vi "Client.vi"() -> ()   [LabVIEW 2019]
uses:
  padrao_tipo_dado.ctl
  padrao_todos_os_dados_ENTRADA.ctl
  padrao_UCM.004.EEL.0300_ENTRADA.ctl
  padrao_UCM.004.EEL.0200_ENTRADA.ctl
  padrao_INTERNO.ctl
  padrao_todos_os_dados_SAIDA.ctl
  padrao_UCM.004.EEL.0300_SAIDA.ctl
  padrao_UCM.004.EEL.0200_SAIDA.ctl
  padrao_enum.ctl
  padrao_TAGS_prioridades_client.ctl
  padrao_dados_cliente_para_server.ctl
  padrao_informacoes_meu_computador.ctl
  <vilib>/Utility/config.llb/NI_LVConfig.lvlib
panel:
  out "Array_TAGS":string[](array[string])
  in  "todos_os_dados_SAIDA":T1
  out "todos_os_dados_ENTRADA":T5
  in  "TAG_para_PDF":string
  in  "Refresh Button":bool
  in  "Seleciona_variaveis_prioridade":bool
  in  "Tipo de Dado":T8 items=["Engenharia", "Puro(mA)"]
  out "Nome_meu_computador":string
  out "Meu IP":string
  out "Status_Comunicação":string
  out "led_indica_comunicacao":bool
  in  "Endereço IP do Server":string(combo)
  in  "[ESC]":bool
  out "Erro":errorcluster
  # "CLIENT"
  # "1) Certifique-se que esse não é o PC Server: Caso for, essa VI não pode rodar nesse computador.\n2) Certifique-se que o Server já esteja rodando:  Caso esteja, você poder rodar essa VI apertando Ctrl+R ou na seta ->\n3) Se não ocorrer nenhum erro, o LED azul irá acender\n4) Coloque o nome do PC caso esteja em branco.\n5) Caso deseje encerrar aperte ESC ou no botão STOP"
  # "Comunicação Via TCP/IP"
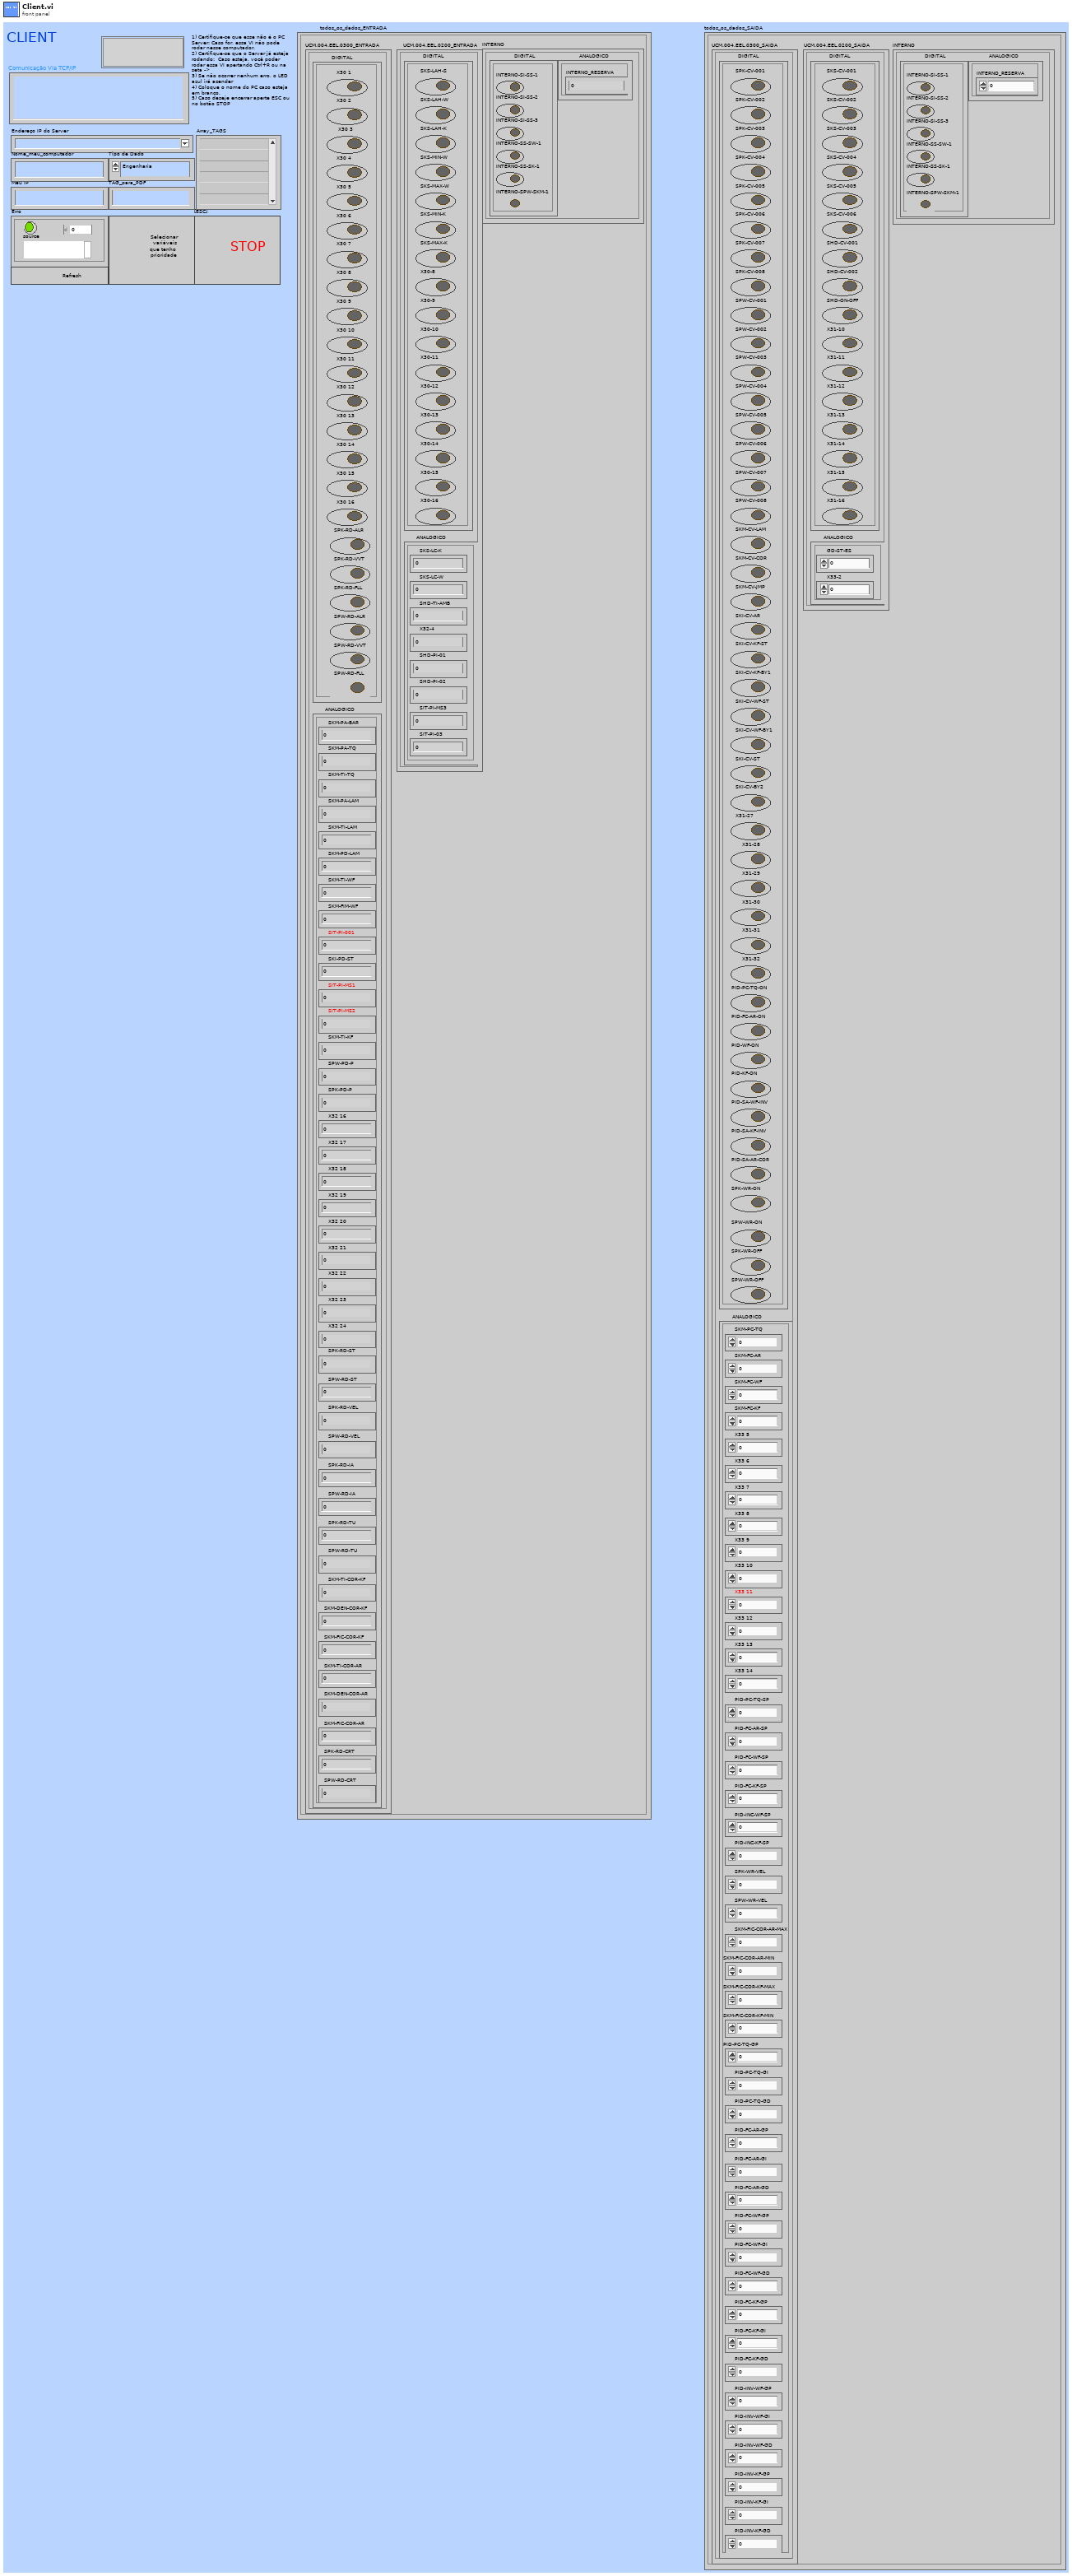
[diagram p1: front panel]
types:
  T1 = typedef "padrao_todos_os_dados_SAIDA.ctl" = cluster{"UCM.004.EEL.0300_SAIDA":T2, "UCM.004.EEL.0200_SAIDA":T3, "INTERNO":T4}
  T2 = typedef "padrao_UCM.004.EEL.0300_SAIDA.ctl" = cluster{"DIGITAL":cluster{"SPK-CV-001":bool, "SPK-CV-002":bool, "SPK-CV-003":bool, "SPK-CV-004":bool, "SPK-CV-005":bool, "SPK-CV-006":bool, "SPK-CV-007":bool, "SPK-CV-008":bool, "SPW-CV-001":bool, "SPW-CV-002":bool, "SPW-CV-003":bool, "SPW-CV-004":bool, "SPW-CV-005":bool, "SPW-CV-006":bool, "SPW-CV-007":bool, "SPW-CV-008":bool, "SKM-CV-LAM":bool, "SKM-CV-COR":bool, "SKM-CV-JMP":bool, "SKI-CV-AR":bool, "SKI-CV-KF-ST":bool, "SKI-CV-KF-BY1":bool, "SKI-CV-WF-ST":bool, "SKI-CV-WF-BY1":bool, "SKI-CV-ST":bool, "SKI-CV-BY2":bool, "X31-27":bool, "X31-28":bool, "X31-29":bool, "X31-30":bool, "X31-31":bool, "X31-32":bool, "PID-PC-TQ-ON":bool, "PID-FC-AR-ON":bool, "PID-WF-ON":bool, "PID-KF-ON":bool, "PID-SA-WF-INV":bool, "PID-SA-KF-INV":bool, "PID-SA-AR-COR":bool, "SPK-WR-ON":bool, "SPW-WR-ON":bool, "SPK-WR-OFF":bool, "SPW-WR-OFF":bool}, "ANALOGICO":cluster{"SKM-PC-TQ":i16, "SKM-FC-AR":i16, "SKM-FC-WF":i16, "SKM-FC-KF":i16, "X33 5":i16, "X33 6":i16, "X33 7":i16, "X33 8":i16, "X33 9":i16, "X33 10":i16, "X33 11":i16, "X33 12":i16, "X33 13":i16, "X33 14":i16, "PID-PC-TQ-SP":i16, "PID-FC-AR-SP":i16, "PID-FC-WF-SP":i16, "PID-FC-KF-SP":i16, "PID-INC-WF-SP":i16, "PID-INC-KF-SP":i16, "SPK-WR-VEL":i32, "SPW-WR-VEL":i32, "SKM-FIC-COR-AR-MAX":dbl, "SKM-FIC-COR-AR-MIN":dbl, "SKM-FIC-COR-KF-MAX":dbl, "SKM-FIC-COR-KF-MIN":dbl, "PID-PC-TQ-GP":dbl, "PID-PC-TQ-GI":dbl, "PID-PC-TQ-GD":dbl, "PID-FC-AR-GP":dbl, "PID-FC-AR-GI":dbl, "PID-FC-AR-GD":dbl, "PID-FC-WF-GP":dbl, "PID-FC-WF-GI":dbl, "PID-FC-WF-GD":dbl, "PID-FC-KF-GP":dbl, "PID-FC-KF-GI":dbl, "PID-FC-KF-GD":dbl, "PID-INV-WF-GP":dbl, "PID-INV-WF-GI":dbl, "PID-INV-WF-GD":dbl, "PID-INV-KF-GP":dbl, "PID-INV-KF-GI":dbl, "PID-INV-KF-GD":dbl}}
  T3 = typedef "padrao_UCM.004.EEL.0200_SAIDA.ctl" = cluster{"DIGITAL":cluster{"SKS-CV-001":bool, "SKS-CV-002":bool, "SKS-CV-003":bool, "SKS-CV-004":bool, "SKS-CV-005":bool, "SKS-CV-006":bool, "SHD-CV-001":bool, "SHD-CV-002":bool, "SHD-ON-OFF":bool, "X31-10":bool, "X31-11":bool, "X31-12":bool, "X31-13":bool, "X31-14":bool, "X31-15":bool, "X31-16":bool}, "ANALOGICO":cluster{"GD-ST-ES":i16, "X33-2":i16}}
  T4 = typedef "padrao_INTERNO.ctl" = cluster{"DIGITAL":cluster{"INTERNO-SI-SS-1":bool, "INTERNO-SI-SS-2":bool, "INTERNO-SI-SS-3":bool, "INTERNO-SS-SW-1":bool, "INTERNO-SS-SK-1":bool, "INTERNO-SPW-SKM-1":bool}, "ANALOGICO":cluster{"INTERNO_RESERVA":dbl}}
  T5 = typedef "padrao_todos_os_dados_ENTRADA.ctl" = cluster{"UCM.004.EEL.0300_ENTRADA":T6, "UCM.004.EEL.0200_ENTRADA":T7, "INTERNO":T4}
  T6 = typedef "padrao_UCM.004.EEL.0300_ENTRADA.ctl" = cluster{"DIGITAL":cluster{"X30 1":bool, "X30 2":bool, "X30 3":bool, "X30 4":bool, "X30 5":bool, "X30 6":bool, "X30 7":bool, "X30 8":bool, "X30 9":bool, "X30 10":bool, "X30 11":bool, "X30 12":bool, "X30 13":bool, "X30 14":bool, "X30 15":bool, "X30 16":bool, "SPK-RD-ALR":bool, "SPK-RD-VVT":bool, "SPK-RD-FLL":bool, "SPW-RD-ALR":bool, "SPW-RD-VVT":bool, "SPW-RD-FLL":bool}, "ANALOGICO":cluster{"SKM-PA-BAR":i16, "SKM-PA-TQ":i16, "SKM-TI-TQ":i16, "SKM-PA-LAM":i16, "SKM-TI-LAM":i16, "SKM-PD-LAM":i16, "SKM-TI-WF":i16, "SKM-FIM-WF":i16, "SIT-PI-001":i16, "SKI-PD-ST":i16, "SIT-PI-MS1":i16, "SIT-PI-MS2":i16, "SKM-TI-KF":i16, "SPW-PD-P":i16, "SPK-PD-P":i16, "X32 16 ":i16, "X32 17":i16, "X32 18":i16, "X32 19":i16, "X32 20":i16, "X32 21":i16, "X32 22":i16, "X32 23":i16, "X32 24":i16, "SPK-RD-ST":i32, "SPW-RD-ST":i32, "SPK-RD-VEL":i32, "SPW-RD-VEL":i32, "SPK-RD-IA":i32, "SPW-RD-IA":i32, "SPK-RD-TU":i32, "SPW-RD-TU":i32, "SKM-TI-COR-KF":dbl, "SKM-DEN-COR-KF":dbl, "SKM-FIC-COR-KF":dbl, "SKM-TI-COR-AR":dbl, "SKM-DEN-COR-AR":dbl, "SPK-RD-CRT":dbl, "SPW-RD-CRT":dbl, "SKM-FIC-COR-AR":dbl}}
  T7 = typedef "padrao_UCM.004.EEL.0200_ENTRADA.ctl" = cluster{"DIGITAL":cluster{"SKS-LAH-S":bool, "SKS-LAH-W":bool, "SKS-LAH-K":bool, "SKS-MIN-W":bool, "SKS-MAX-W":bool, "SKS-MIN-K":bool, "SKS-MAX-K":bool, "X30-8":bool, "X30-9":bool, "X30-10":bool, "X30-11":bool, "X30-12":bool, "X30-13":bool, "X30-14":bool, "X30-15":bool, "X30-16":bool}, "ANALOGICO":cluster{"SKS-LC-K":i16, "SKS-LC-W":i16, "SHD-TI-AMB":i16, "X32-4":i16, "SHD-PI-01":i16, "SHD-PI-02":i16, "SIT-PI-MS3":i16, "SIT-PI-03":i16}}
  T8 = typedef "padrao_tipo_dado.ctl" = u16
  T9 = typedef "padrao_TAGS_prioridades_client.ctl" = cluster{"TAG":string, "Tenho\nPrioridade?":bool}[]
  T10 = typedef "padrao_enum.ctl" = enum16{"open-conection ", "data", "check-status", "Inicio"}
  T11 = typedef "NI_LVConfig.lvlib/Config Data RefNum.ctl" = refnum<k1>
  T12 = typedef "padrao_informacoes_meu_computador.ctl" = cluster{"Nome_computador":string, "IP_meu_computador":string, "Tipo de Dado":T8}
  T13 = typedef "padrao_dados_cliente_para_server.ctl" = cluster{"todos_os_dados_saida":T1, "informacoes_meu_PC":T12, "padrao_prioridade_TAGs":T9}
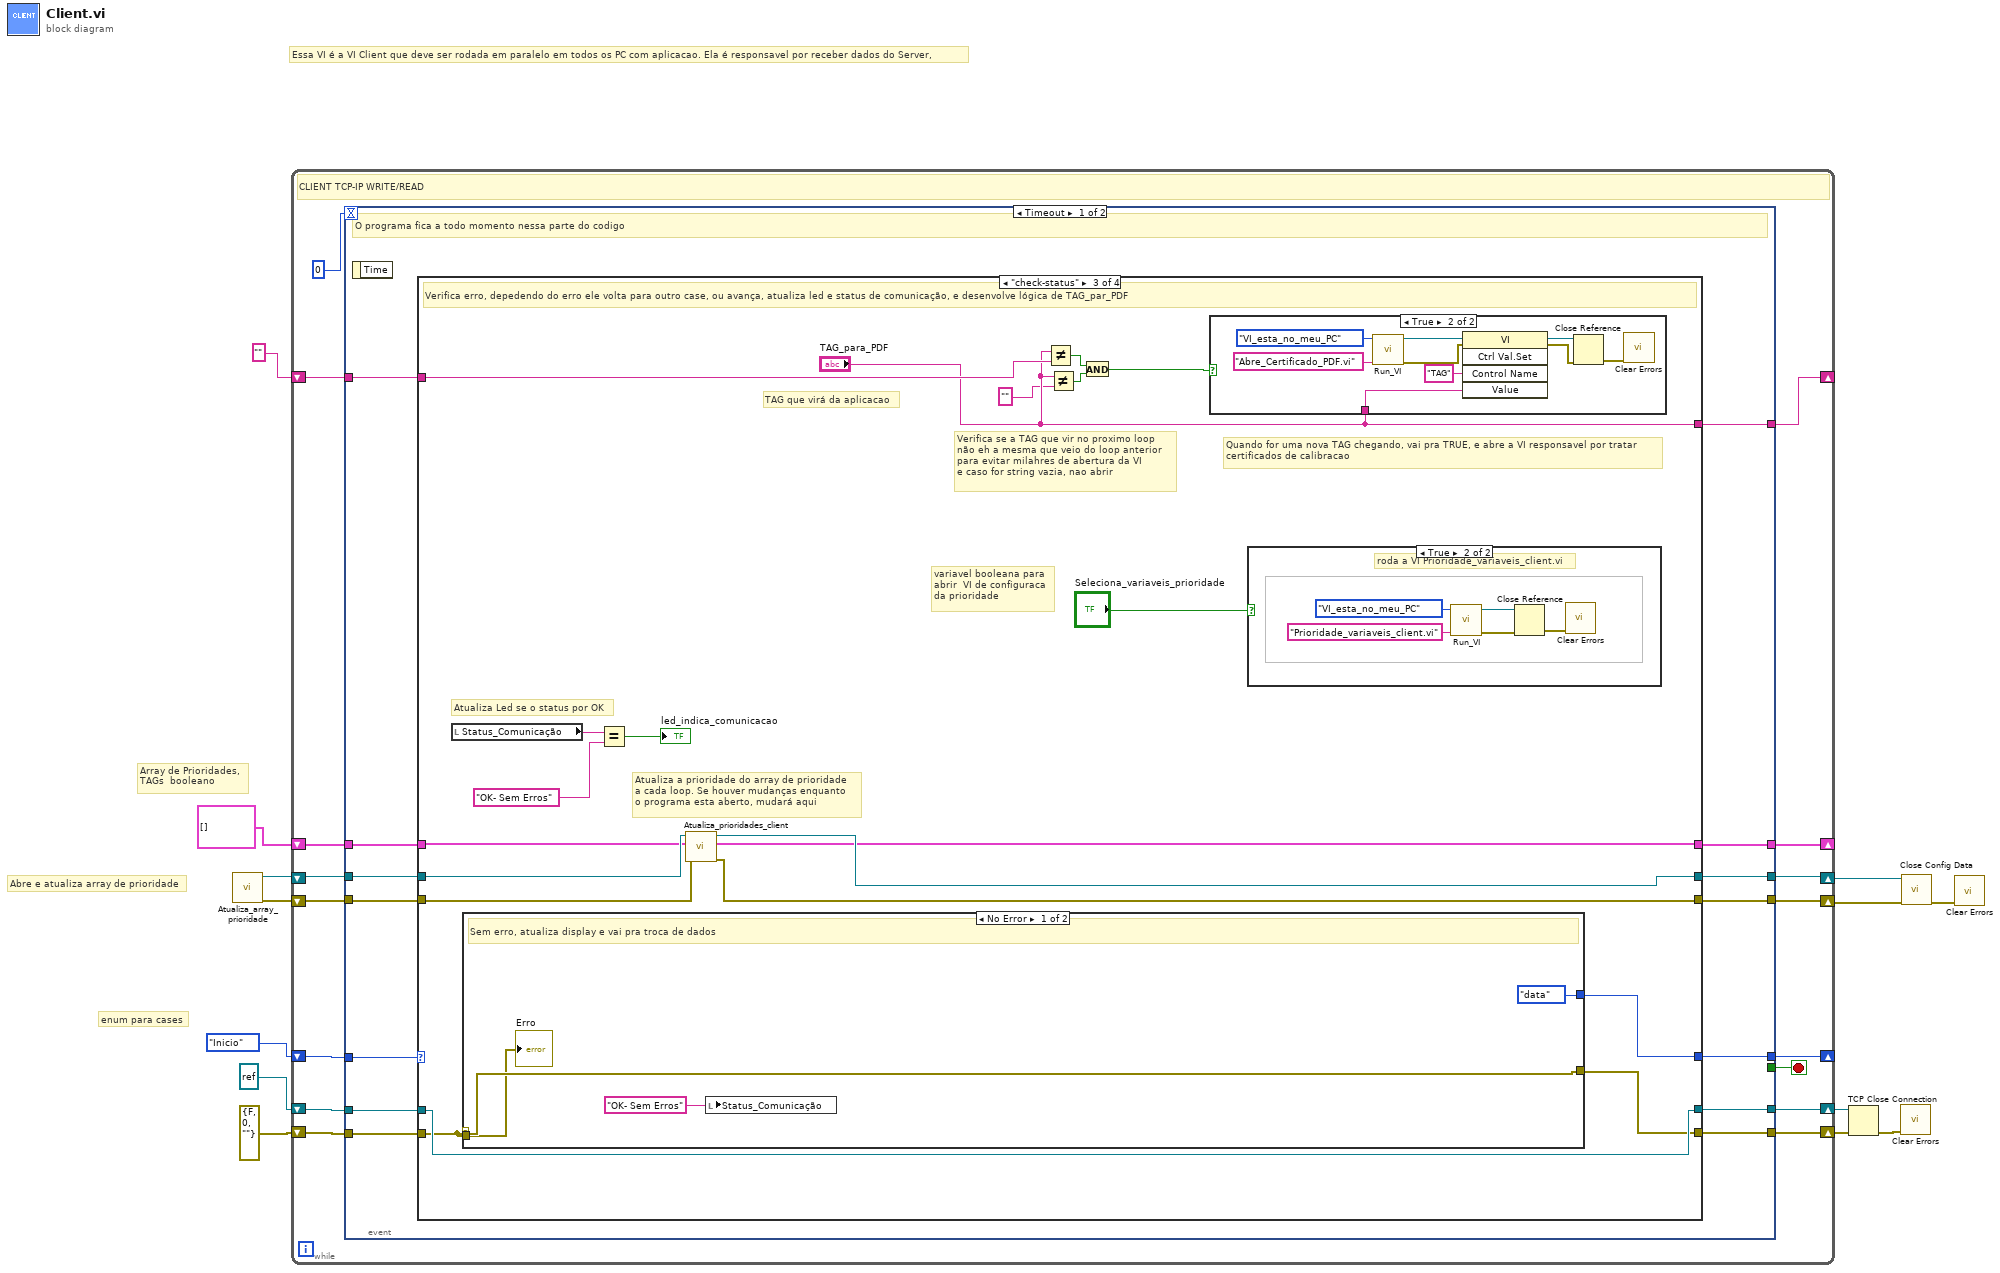
[diagram p0: block diagram]
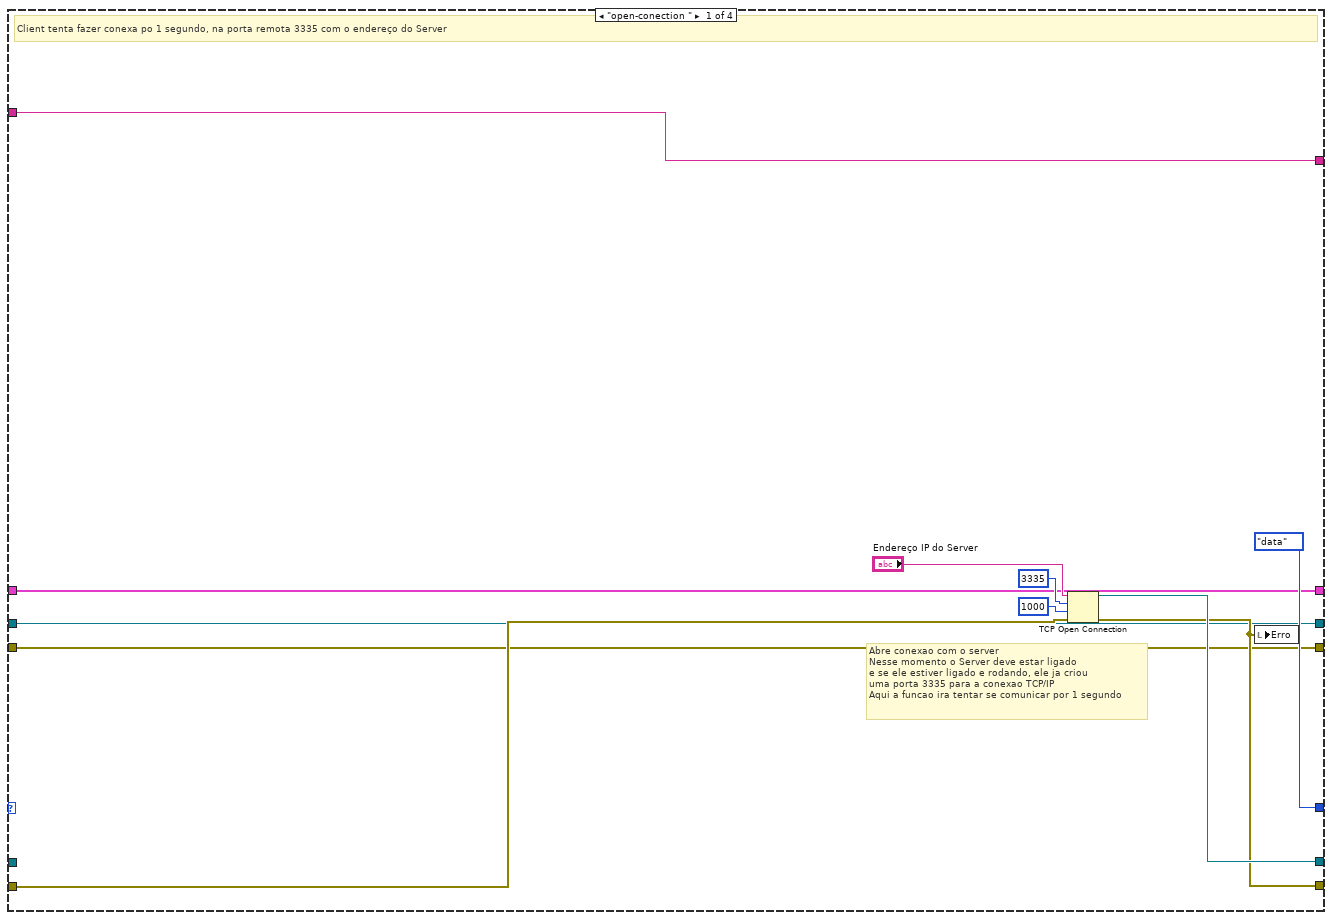
[diagram p2: hidden frame]
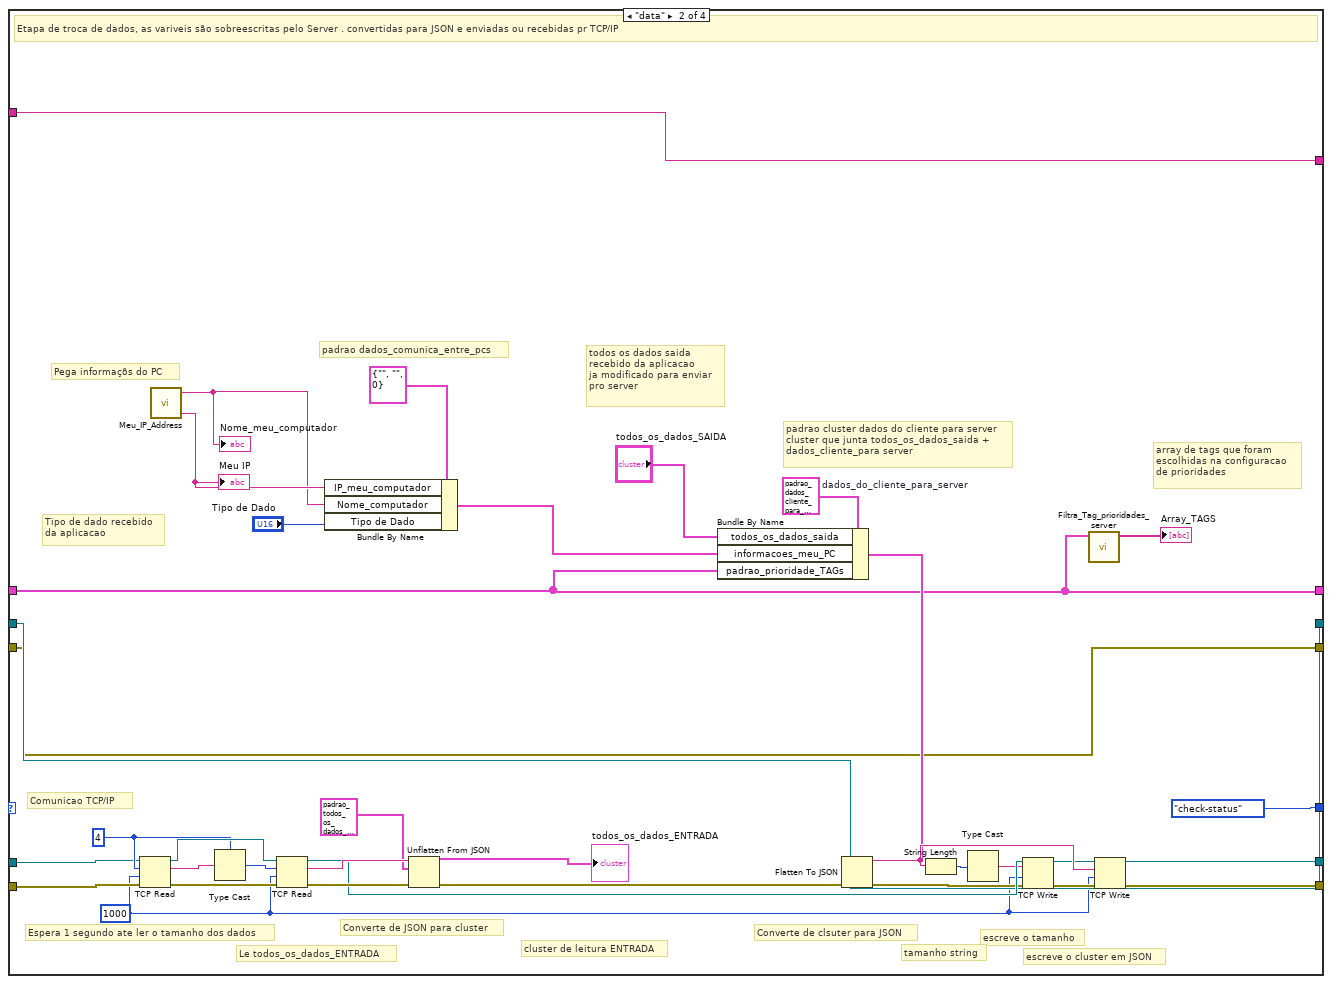
[diagram p3: hidden frame]
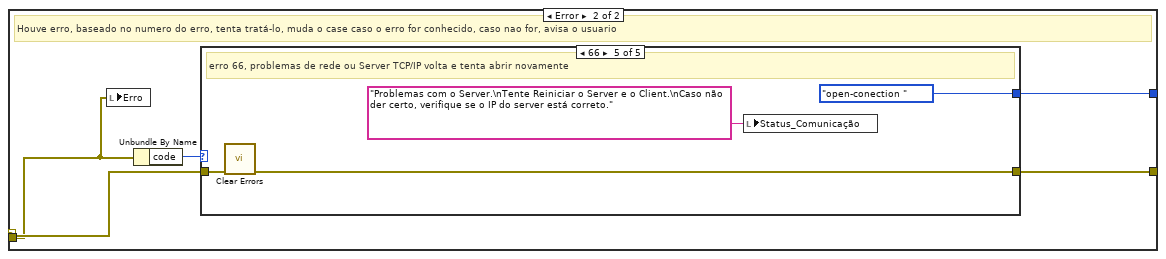
[diagram p6: hidden frame]
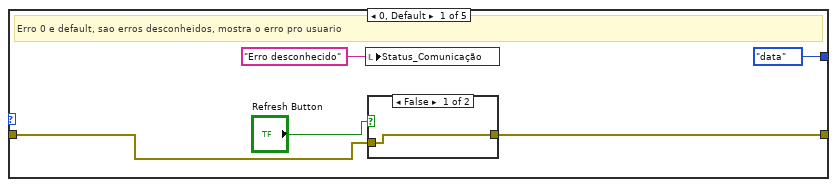
[diagram p7: hidden frame]
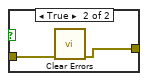
[diagram p8: hidden frame]
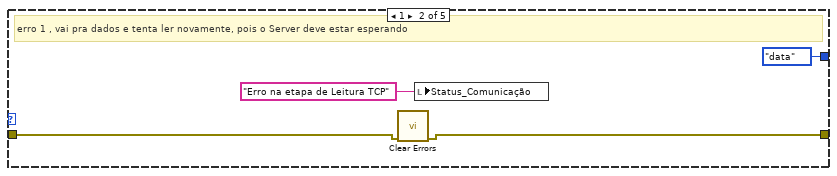
[diagram p9: hidden frame]
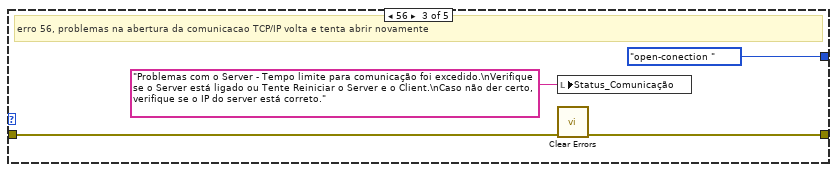
[diagram p10: hidden frame]
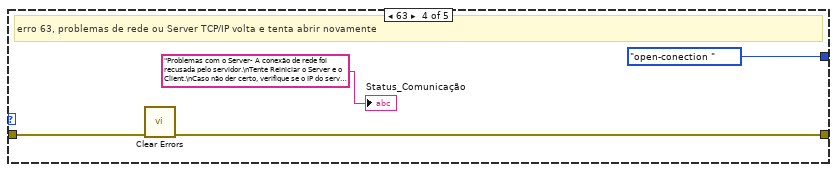
[diagram p11: hidden frame]
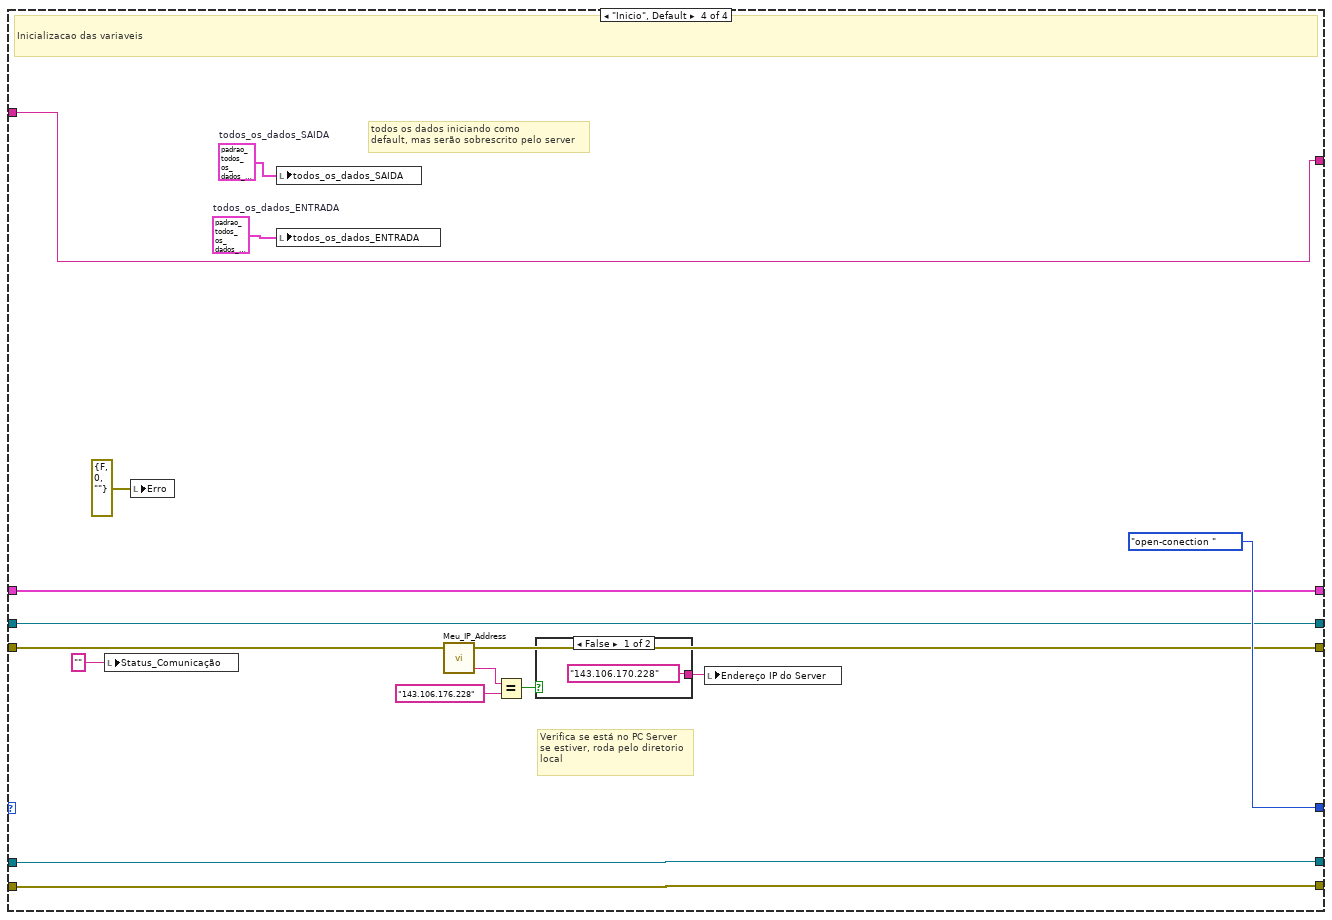
[diagram p12: hidden frame]
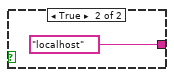
[diagram p13: hidden frame]
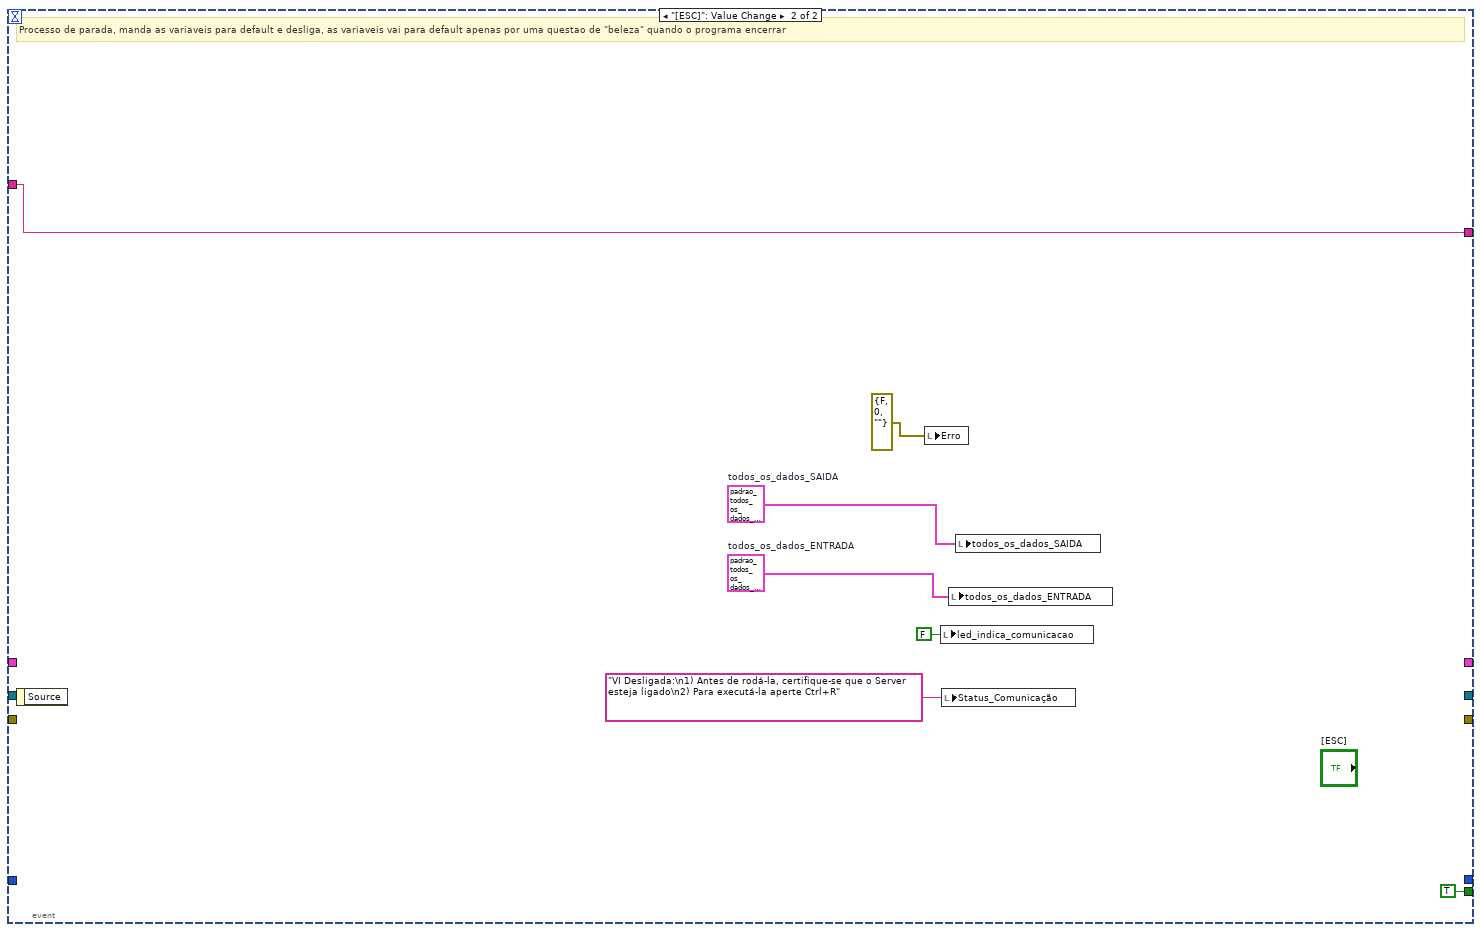
[diagram p14: hidden frame]
diagram:
  # "Array de Prioridades,\nTAGs  booleano"
  # "enum para cases"
  # "Abre e atualiza array de prioridade"
  # "Essa VI é a VI Client que deve ser rodada em paralelo em todos os PC com aplicacao. Ela é responsavel por receber dados do Server,"
  n1 = call "Atualiza_array_prioridade.vi"() -> ("error out"=w1:errorcluster, "refnum"=w2:T11)  [unwired: 10 in]
  n2 = while {
    shift-right: [w26] -> w9
    shift-left: errorcluster {"status"=FALSE, "code"=0, "source"=""} ("error constant") -> [w27]
    shift-right: [w28] -> _
    shift-left: padrao_enum."Inicio" ("Enum") -> [w29]
    shift-right: [w25] -> w10
    shift-left: refnum<k5> refnum ("connection ID") -> [w24]
    shift-right: [w19] -> w6
    shift-left: w2 -> [w21]
    shift-right: [w18] -> w7
    shift-left: w1 -> [w20]
    shift-right: [w16] -> _
    shift-left: T9 [] ("padrao_prioridade_TAGs") -> [w17]
    shift-right: [w14] -> _
    shift-left: "" ("y") -> [w15]
    stop <- w22 stop-if-true
    # "CLIENT TCP-IP WRITE/READ"
    n3 = event shown="[0] Timeout" {
      selector: _ -> [_ _]
      dyn-events: _ -> [_ _]
      timeout: 0 -> [_ _]
      tunnel: w29 -> [w43 _]
      tunnel: [w42 _] -> w28
      tunnel: w27 -> [w41 _]
      tunnel: [w40 _] -> w26
      tunnel: [w39 _] -> w25
      tunnel: w24 -> [w38 _]
      tunnel: [_ TRUE ("[ESC]")] -> w22
      tunnel: w21 -> [w37 _]
      tunnel: w20 -> [w36 _]
      tunnel: [w35 _] -> w19
      tunnel: [w34 _] -> w18
      tunnel: w17 -> [w33 _]
      tunnel: [w32 _] -> w16
      tunnel: w15 -> [w31 w175]
      tunnel: [w30 w175] -> w14
      event Timeout {
        # "O programa fica a todo momento nessa parte do codigo"
        n4 = event-data() -> ()  [unwired: 1 in, 1 out]
        n5 = case shown="\"check-status\"" w43 {
          tunnel: [padrao_enum."data" ("Enum") padrao_enum."check-status" ("Enum") w107 padrao_enum."open-conection " ("Enum")] -> w42
          tunnel: w41 -> [w53 w81 w108 w170]
          tunnel: [w50 w71 w109 w170] -> w40
          tunnel: [w52 w72 w110 w172] -> w39
          tunnel: w38 -> [_ w82 w110 w172]
          tunnel: w37 -> [w47 w64 w103 w163]
          tunnel: w36 -> [w46 w63 w102 w162]
          tunnel: [w47 w64 w101 w163] -> w35
          tunnel: [w46 w63 w100 w162] -> w34
          tunnel: w33 -> [w45 w56 w98 w161]
          tunnel: [w45 w56 w99 w161] -> w32
          tunnel: w31 -> [w44 w57 w97 w158]
          tunnel: [w44 w57 "TAG_para_PDF" w158] -> w30
          frame "open-conection " {
            # "Abre conexao com o server\nNesse momento o Server deve estar ligado\ne se ele estiver ligado e rodando, ele ja criou\numa porta 3335 para a conexao TCP/IP\nAqui a funcao ira tentar se comunicar por 1 segundo"
            # "Client tenta fazer conexa po 1 segundo, na porta remota 3335 com o endereço do Server"
            n6 = TCP Open Connection(address="Endereço IP do Server", remote port or service name=u16 3335, timeout ms (60000)=1000, error in (no error)=w53) -> (connection ID=w52:refnum<k5>, error out=w50:errorcluster)  [unwired: 1 in]
            n7 = local write "Erro"(w50) -> ()
          }
          frame "data" {
            w58 = 1000 ("timeout ms (25000)")
            w70 = T13 {"todos_os_dados_saida"={"UCM.004.EEL.0300_SAIDA"={"DIGITAL"={"SPK-CV-001"=FALSE, "SPK-CV-002"=FALSE, "SPK-CV-003"=FALSE, "SPK-CV-004"=FALSE, "SPK-CV-005"=FALSE, "SPK-CV-006"=FALSE, "SPK-CV-007"=FALSE, "SPK-CV-008"=FALSE, "SPW-CV-001"=FALSE, "SPW-CV-002"=FALSE, "SPW-CV-003"=FALSE, "SPW-CV-004"=FALSE, "SPW-CV-005"=FALSE, "SPW-CV-006"=FALSE, "SPW-CV-007"=FALSE, "SPW-CV-008"=FALSE, "SKM-CV-LAM"=FALSE, "SKM-CV-COR"=FALSE, "SKM-CV-JMP"=FALSE, "SKI-CV-AR"=FALSE, "SKI-CV-KF-ST"=FALSE, "SKI-CV-KF-BY1"=FALSE, "SKI-CV-WF-ST"=FALSE, "SKI-CV-WF-BY1"=FALSE, "SKI-CV-ST"=FALSE, "SKI-CV-BY2"=FALSE, "X31-27"=FALSE, "X31-28"=FALSE, "X31-29"=FALSE, "X31-30"=FALSE, "X31-31"=FALSE, "X31-32"=FALSE, "PID-PC-TQ-ON"=FALSE, "PID-FC-AR-ON"=FALSE, "PID-WF-ON"=FALSE, "PID-KF-ON"=FALSE, "PID-SA-WF-INV"=FALSE, "PID-SA-KF-INV"=FALSE, "PID-SA-AR-COR"=FALSE, "SPK-WR-ON"=FALSE, "SPW-WR-ON"=FALSE, "SPK-WR-OFF"=FALSE, "SPW-WR-OFF"=FALSE}, "ANALOGICO"={"SKM-PC-TQ"=0, "SKM-FC-AR"=0, "SKM-FC-WF"=0, "SKM-FC-KF"=0, "X33 5"=0, "X33 6"=0, "X33 7"=0, "X33 8"=0, "X33 9"=0, "X33 10"=0, "X33 11"=0, "X33 12"=0, "X33 13"=0, "X33 14"=0, "PID-PC-TQ-SP"=0, "PID-FC-AR-SP"=0, "PID-FC-WF-SP"=0, "PID-FC-KF-SP"=0, "PID-INC-WF-SP"=0, "PID-INC-KF-SP"=0, "SPK-WR-VEL"=0, "SPW-WR-VEL"=0, "SKM-FIC-COR-AR-MAX"=0.0, "SKM-FIC-COR-AR-MIN"=0.0, "SKM-FIC-COR-KF-MAX"=0.0, "SKM-FIC-COR-KF-MIN"=0.0, "PID-PC-TQ-GP"=0.0, "PID-PC-TQ-GI"=0.0, "PID-PC-TQ-GD"=0.0, "PID-FC-AR-GP"=0.0, "PID-FC-AR-GI"=0.0, "PID-FC-AR-GD"=0.0, "PID-FC-WF-GP"=0.0, "PID-FC-WF-GI"=0.0, "PID-FC-WF-GD"=0.0, "PID-FC-KF-GP"=0.0, "PID-FC-KF-GI"=0.0, "PID-FC-KF-GD"=0.0, "PID-INV-WF-GP"=0.0, "PID-INV-WF-GI"=0.0, "PID-INV-WF-GD"=0.0, "PID-INV-KF-GP"=0.0, "PID-INV-KF-GI"=0.0, "PID-INV-KF-GD"=0.0}}, "UCM.004.EEL.0200_SAIDA"={"DIGITAL"={"SKS-CV-001"=FALSE, "SKS-CV-002"=FALSE, "SKS-CV-003"=FALSE, "SKS-CV-004"=FALSE, "SKS-CV-005"=FALSE, "SKS-CV-006"=FALSE, "SHD-CV-001"=FALSE, "SHD-CV-002"=FALSE, "SHD-ON-OFF"=FALSE, "X31-10"=FALSE, "X31-11"=FALSE, "X31-12"=FALSE, "X31-13"=FALSE, "X31-14"=FALSE, "X31-15"=FALSE, "X31-16"=FALSE}, "ANALOGICO"={"GD-ST-ES"=0, "X33-2"=0}}, "INTERNO"={"DIGITAL"={"INTERNO-SI-SS-1"=FALSE, "INTERNO-SI-SS-2"=FALSE, "INTERNO-SI-SS-3"=FALSE, "INTERNO-SS-SW-1"=FALSE, "INTERNO-SS-SK-1"=FALSE, "INTERNO-SPW-SKM-1"=FALSE}, "ANALOGICO"={"INTERNO_RESERVA"=0.0}}}, "informacoes_meu_PC"={"Nome_computador"="", "IP_meu_computador"="", "Tipo de Dado"=0}, "padrao_prioridade_TAGs"=[]}  # dados_do_cliente_para_server
            w83 = 4
            # "array de tags que foram\nescolhidas na configuracao\nde prioridades"
            # "padrao cluster dados do cliente para server\ncluster que junta todos_os_dados_saida +\ndados_cliente_para server"
            # "todos os dados saida\nrecebido da aplicacao\nja modificado para enviar\npro server"
            # "padrao dados_comunica_entre_pcs"
            # "Tipo de dado recebido\nda aplicacao"
            # "Pega informaçõs do PC"
            # "escreve o cluster em JSON"
            # "escreve o tamanho"
            # "tamanho string"
            # "Converte de clsuter para JSON"
            # "cluster de leitura ENTRADA"
            # "Converte de JSON para cluster"
            # "Le todos_os_dados_ENTRADA"
            # "Espera 1 segundo ate ler o tamanho dos dados"
            # "Comunicao TCP/IP"
            # "Etapa de troca de dados, as variveis são sobreescritas pelo Server . convertidas para JSON e enviadas ou recebidas pr TCP/IP"
            n8 = TCP Read(connection ID=w82, bytes to read=w83, error in (no error)=w81, 9:w58) -> (connection ID out=w87:refnum<k5>, data out=w89:string, error out=w85:errorcluster)  [unwired: 1 out]
            n9 = call "Meu_IP_Address.vi"() -> ("Meu IP"=w68:string, "Nome computador"=w62:string)  [unwired: 4 in]
            "Nome_meu_computador" <- w62
            "Meu IP" <- w68
            n10 = Type Cast(type=w83, x=w89) -> (*(type *) &x=w88:i32)
            n11 = TCP Read(connection ID=w87, bytes to read=w88, error in (no error)=w85, 9:w58) -> (connection ID out=w80:refnum<k5>, data out=w86:string, error out=w84:errorcluster)  [unwired: 1 in]
            n12 = Bundle By Name(cluster=T12 {"Nome_computador"="", "IP_meu_computador"="", "Tipo de Dado"=0} ("informacoes_meu_PC"), "IP_meu_computador"=w68, "Nome_computador"=w62, "Tipo de Dado"="Tipo de Dado") -> (w67:T12)
            n13 = Unflatten From JSON(JSON string=w86, type and defaults=T5 {"UCM.004.EEL.0300_ENTRADA"={"DIGITAL"={"X30 1"=FALSE, "X30 2"=FALSE, "X30 3"=FALSE, "X30 4"=FALSE, "X30 5"=FALSE, "X30 6"=FALSE, "X30 7"=FALSE, "X30 8"=FALSE, "X30 9"=FALSE, "X30 10"=FALSE, "X30 11"=FALSE, "X30 12"=FALSE, "X30 13"=FALSE, "X30 14"=FALSE, "X30 15"=FALSE, "X30 16"=FALSE, "SPK-RD-ALR"=FALSE, "SPK-RD-VVT"=FALSE, "SPK-RD-FLL"=FALSE, "SPW-RD-ALR"=FALSE, "SPW-RD-VVT"=FALSE, "SPW-RD-FLL"=FALSE}, "ANALOGICO"={"SKM-PA-BAR"=0, "SKM-PA-TQ"=0, "SKM-TI-TQ"=0, "SKM-PA-LAM"=0, "SKM-TI-LAM"=0, "SKM-PD-LAM"=0, "SKM-TI-WF"=0, "SKM-FIM-WF"=0, "SIT-PI-001"=0, "SKI-PD-ST"=0, "SIT-PI-MS1"=0, "SIT-PI-MS2"=0, "SKM-TI-KF"=0, "SPW-PD-P"=0, "SPK-PD-P"=0, "X32 16 "=0, "X32 17"=0, "X32 18"=0, "X32 19"=0, "X32 20"=0, "X32 21"=0, "X32 22"=0, "X32 23"=0, "X32 24"=0, "SPK-RD-ST"=0, "SPW-RD-ST"=0, "SPK-RD-VEL"=0, "SPW-RD-VEL"=0, "SPK-RD-IA"=0, "SPW-RD-IA"=0, "SPK-RD-TU"=0, "SPW-RD-TU"=0, "SKM-TI-COR-KF"=0.0, "SKM-DEN-COR-KF"=0.0, "SKM-FIC-COR-KF"=0.0, "SKM-TI-COR-AR"=0.0, "SKM-DEN-COR-AR"=0.0, "SPK-RD-CRT"=0.0, "SPW-RD-CRT"=0.0, "SKM-FIC-COR-AR"=0.0}}, "UCM.004.EEL.0200_ENTRADA"={"DIGITAL"={"SKS-LAH-S"=FALSE, "SKS-LAH-W"=FALSE, "SKS-LAH-K"=FALSE, "SKS-MIN-W"=FALSE, "SKS-MAX-W"=FALSE, "SKS-MIN-K"=FALSE, "SKS-MAX-K"=FALSE, "X30-8"=FALSE, "X30-9"=FALSE, "X30-10"=FALSE, "X30-11"=FALSE, "X30-12"=FALSE, "X30-13"=FALSE, "X30-14"=FALSE, "X30-15"=FALSE, "X30-16"=FALSE}, "ANALOGICO"={"SKS-LC-K"=0, "SKS-LC-W"=0, "SHD-TI-AMB"=0, "X32-4"=0, "SHD-PI-01"=0, "SHD-PI-02"=0, "SIT-PI-MS3"=0, "SIT-PI-03"=0}}, "INTERNO"={"DIGITAL"={"INTERNO-SI-SS-1"=FALSE, "INTERNO-SI-SS-2"=FALSE, "INTERNO-SI-SS-3"=FALSE, "INTERNO-SS-SW-1"=FALSE, "INTERNO-SS-SK-1"=FALSE, "INTERNO-SPW-SKM-1"=FALSE}, "ANALOGICO"={"INTERNO_RESERVA"=0.0}}} ("todos_os_dados_ENTRADA"), error in (no error)=w84) -> (value=→"todos_os_dados_ENTRADA":T5, error out=w75:errorcluster)  [unwired: 4 in]
            n14 = Bundle By Name(cluster=w70, "todos_os_dados_saida"="todos_os_dados_SAIDA", "informacoes_meu_PC"=w67, "padrao_prioridade_TAGs"=w56) -> (w69:T13)
            n15 = Flatten To JSON(anything=w69, error in (no error)=w75) -> (JSON string=w78:string, 11:w76:errorcluster)  [unwired: 1 in]
            n16 = String Length(string=w78) -> (length=w77:i32)
            n17 = Type Cast(x=w77) -> (*(type *) &x=w79:string)  [unwired: 1 in]
            n18 = TCP Write(connection ID=w80, data in=w79, error in (no error)=w76, 9:w58) -> (connection ID out=w74:refnum<k5>, error out=w73:errorcluster)  [unwired: 1 out]
            n19 = call "Filtra_Tag_prioridades_server.vi"("padrao_TAGS_prioridade_client"=w56) -> ("TAGs prioridade"=→"Array_TAGS":string[])  [unwired: 10 in]
            n20 = TCP Write(connection ID=w74, data in=w78, error in (no error)=w73, 9:w58) -> (connection ID out=w72:refnum<k5>, error out=w71:errorcluster)  [unwired: 1 out]
          }
          frame "check-status" {
            # "variavel booleana para \nabrir  VI de configuraca\nda prioridade"
            # "Quando for uma nova TAG chegando, vai pra TRUE, e abre a VI responsavel por tratar\ncertificados de calibracao"
            # "Verifica se a TAG que vir no proximo loop\nnão eh a mesma que veio do loop anterior\npara evitar milahres de abertura da VI\ne caso for string vazia, nao abrir"
            # "TAG que virá da aplicacao"
            # "Atualiza a prioridade do array de prioridade\na cada loop. Se houver mudanças enquanto\no programa esta aberto, mudará aqui"
            # "Atualiza Led se o status por OK"
            # "Verifica erro, depedendo do erro ele volta para outro case, ou avança, atualiza led e status de comunicação, e desenvolve lógica de TAG_par_PDF"
            n21 = local read "Status_Comunicação"() -> (w104:string)
            n22 = case shown="No Error" w108 {
              selector: w108 -> [w128 w132]
              tunnel: [w128 w131] -> w109
              tunnel: w108 -> [w127 w129]
              tunnel: [padrao_enum."data" ("Enum") w130] -> w107
              frame No Error {
                # "Sem erro, atualiza display e vai pra troca de dados"
                n23 = local write "Status_Comunicação"("OK- Sem Erros" ("Status")) -> ()
                "Erro" <- w127
              }
              frame Error {
                # "Houve erro, baseado no numero do erro, tenta tratá-lo, muda o case caso o erro for conhecido, caso nao for, avisa o usuario"
                n24 = local write "Erro"(w129) -> ()
                n25 = Unbundle By Name(w129) -> ("code"=w133:i32)
                n26 = case shown="66" w133 {
                  tunnel: w132 -> [w135 w144 w149 w153 w157]
                  tunnel: [w134 w143 w148 w152 w156] -> w131
                  tunnel: [padrao_enum."data" ("Enum") padrao_enum."data" ("Enum") padrao_enum."open-conection " ("Enum") padrao_enum."open-conection " ("Enum") padrao_enum."open-conection " ("Enum")] -> w130
                  frame 0, Default {
                    # "Erro 0 e default, sao erros desconheidos, mostra o erro pro usuario"
                    n27 = local write "Status_Comunicação"("Erro desconhecido" ("status")) -> ()
                    n28 = case shown="False" "Refresh Button" {
                      tunnel: w135 -> [w139 w141]
                      tunnel: [w139 w140] -> w134
                      frame False {
                      }
                      frame True {
                        n29 = call <vilib>:"Clear Errors.vi"("error in (no error)"=w141) -> ("error out"=w140:errorcluster)  [unwired: 5 in, 1 out]
                      }
                    }
                  }
                  frame 1 {
                    # "erro 1 , vai pra dados e tenta ler novamente, pois o Server deve estar esperando"
                    n30 = call <vilib>:"Clear Errors.vi"("error in (no error)"=w144) -> ("error out"=w143:errorcluster)  [unwired: 5 in, 1 out]
                    n31 = local write "Status_Comunicação"("Erro na etapa de Leitura TCP" ("status")) -> ()
                  }
                  frame 56 {
                    # "erro 56, problemas na abertura da comunicacao TCP/IP volta e tenta abrir novamente"
                    n32 = local write "Status_Comunicação"("Problemas com o Server - Tempo limite para comunicação foi excedido.\nVerifique se o Server está ligado ou Tente Reiniciar o Server e o Client.\nCaso não der certo, verifique se o IP do server está correto." ("Status")) -> ()
                    n33 = call <vilib>:"Clear Errors.vi"("error in (no error)"=w149) -> ("error out"=w148:errorcluster)  [unwired: 5 in, 1 out]
                  }
                  frame 63 {
                    # "erro 63, problemas de rede ou Server TCP/IP volta e tenta abrir novamente"
                    n34 = call <vilib>:"Clear Errors.vi"("error in (no error)"=w153) -> ("error out"=w152:errorcluster)  [unwired: 5 in, 1 out]
                    "Status_Comunicação" <- "Problemas com o Server- A conexão de rede foi recusada pelo servidor.\nTente Reiniciar o Server e o Client.\nCaso não der certo, verifique se o IP do server está correto." ("Status")
                  }
                  frame 66 {
                    # "erro 66, problemas de rede ou Server TCP/IP volta e tenta abrir novamente"
                    n35 = call <vilib>:"Clear Errors.vi"("error in (no error)"=w157) -> ("error out"=w156:errorcluster)  [unwired: 5 in, 1 out]
                    n36 = local write "Status_Comunicação"("Problemas com o Server.\nTente Reiniciar o Server e o Client.\nCaso não der certo, verifique se o IP do server está correto." ("Status")) -> ()
                  }
                }
              }
            }
            n37 = Equal?(x=w104, y="OK- Sem Erros" ("Status")) -> (x = y?=→"led_indica_comunicacao":bool)
            n38 = call "Atualiza_prioridades_client.vi"("error in"=w102, "padrao_prioridade_TAGs_entrada"=w98, "refnum in"=w103) -> ("error out"=w100:errorcluster, "padrao_prioridade_TAGs_saida"=w99:T9, "refnum out"=w101:T11)  [unwired: 6 in]
            n39 = Not Equal?(x="TAG_para_PDF", y=w97) -> (x != y?=w94:bool)
            n40 = Not Equal?(x="TAG_para_PDF", y="") -> (x != y?=w93:bool)
            n41 = And(x=w94, y=w93) -> (x .and. y?=w92:bool)
            n42 = case shown="True" w92 {
              tunnel: "TAG_para_PDF" -> [_ w116]
              frame False {
              }
              frame True {
                n43 = call "Run_VI.vi"("Nome.vi"="Abre_Certificado_PDF.vi", "Origem_VI"=enum16{"VI_esta_no_meu_PC", "VI_esta_na_rede"}."VI_esta_no_meu_PC") -> ("error out"=w119:errorcluster, "reference out"=w122:refnum<vi>)  [unwired: 8 in]
                n44 = invoke class="VI" method="Ctrl Val.Set"(reference=w122, error in=w119, "Control Name"="TAG", "Value"=w116) -> (reference out=w121:refnum<vi>, error out=w120:errorcluster)  [unwired: 1 in, 3 out]
                n45 = Close Reference(reference=w121, error in (no error)=w120) -> (error out=w123:errorcluster)
                n46 = call <vilib>:"Clear Errors.vi"("error in (no error)"=w123) -> ()  [unwired: 5 in, 2 out]
              }
            }
            n47 = case shown="True" "Seleciona_variaveis_prioridade" {
              frame False {
              }
              frame True {
                # "roda a VI Prioridade_variaveis_client.vi"
                n48 = call "Run_VI.vi"("Nome.vi"="Prioridade_variaveis_client.vi", "Origem_VI"=enum16{"VI_esta_no_meu_PC", "VI_esta_na_rede"}."VI_esta_no_meu_PC") -> ("error out"=w114:errorcluster, "reference out"=w115:refnum<vi>)  [unwired: 8 in]
                n49 = Close Reference(reference=w115, error in (no error)=w114) -> (error out=w113:errorcluster)
                n50 = call <vilib>:"Clear Errors.vi"("error in (no error)"=w113) -> ()  [unwired: 5 in, 2 out]
              }
            }
          }
          frame "Inicio", Default {
            w159 = T5 {"UCM.004.EEL.0300_ENTRADA"={"DIGITAL"={"X30 1"=FALSE, "X30 2"=FALSE, "X30 3"=FALSE, "X30 4"=FALSE, "X30 5"=FALSE, "X30 6"=FALSE, "X30 7"=FALSE, "X30 8"=FALSE, "X30 9"=FALSE, "X30 10"=FALSE, "X30 11"=FALSE, "X30 12"=FALSE, "X30 13"=FALSE, "X30 14"=FALSE, "X30 15"=FALSE, "X30 16"=FALSE, "SPK-RD-ALR"=FALSE, "SPK-RD-VVT"=FALSE, "SPK-RD-FLL"=FALSE, "SPW-RD-ALR"=FALSE, "SPW-RD-VVT"=FALSE, "SPW-RD-FLL"=FALSE}, "ANALOGICO"={"SKM-PA-BAR"=0, "SKM-PA-TQ"=0, "SKM-TI-TQ"=0, "SKM-PA-LAM"=0, "SKM-TI-LAM"=0, "SKM-PD-LAM"=0, "SKM-TI-WF"=0, "SKM-FIM-WF"=0, "SIT-PI-001"=0, "SKI-PD-ST"=0, "SIT-PI-MS1"=0, "SIT-PI-MS2"=0, "SKM-TI-KF"=0, "SPW-PD-P"=0, "SPK-PD-P"=0, "X32 16 "=0, "X32 17"=0, "X32 18"=0, "X32 19"=0, "X32 20"=0, "X32 21"=0, "X32 22"=0, "X32 23"=0, "X32 24"=0, "SPK-RD-ST"=0, "SPW-RD-ST"=0, "SPK-RD-VEL"=0, "SPW-RD-VEL"=0, "SPK-RD-IA"=0, "SPW-RD-IA"=0, "SPK-RD-TU"=0, "SPW-RD-TU"=0, "SKM-TI-COR-KF"=0.0, "SKM-DEN-COR-KF"=0.0, "SKM-FIC-COR-KF"=0.0, "SKM-TI-COR-AR"=0.0, "SKM-DEN-COR-AR"=0.0, "SPK-RD-CRT"=0.0, "SPW-RD-CRT"=0.0, "SKM-FIC-COR-AR"=0.0}}, "UCM.004.EEL.0200_ENTRADA"={"DIGITAL"={"SKS-LAH-S"=FALSE, "SKS-LAH-W"=FALSE, "SKS-LAH-K"=FALSE, "SKS-MIN-W"=FALSE, "SKS-MAX-W"=FALSE, "SKS-MIN-K"=FALSE, "SKS-MAX-K"=FALSE, "X30-8"=FALSE, "X30-9"=FALSE, "X30-10"=FALSE, "X30-11"=FALSE, "X30-12"=FALSE, "X30-13"=FALSE, "X30-14"=FALSE, "X30-15"=FALSE, "X30-16"=FALSE}, "ANALOGICO"={"SKS-LC-K"=0, "SKS-LC-W"=0, "SHD-TI-AMB"=0, "X32-4"=0, "SHD-PI-01"=0, "SHD-PI-02"=0, "SIT-PI-MS3"=0, "SIT-PI-03"=0}}, "INTERNO"={"DIGITAL"={"INTERNO-SI-SS-1"=FALSE, "INTERNO-SI-SS-2"=FALSE, "INTERNO-SI-SS-3"=FALSE, "INTERNO-SS-SW-1"=FALSE, "INTERNO-SS-SK-1"=FALSE, "INTERNO-SPW-SKM-1"=FALSE}, "ANALOGICO"={"INTERNO_RESERVA"=0.0}}}  # todos_os_dados_ENTRADA
            w160 = T1 {"UCM.004.EEL.0300_SAIDA"={"DIGITAL"={"SPK-CV-001"=FALSE, "SPK-CV-002"=FALSE, "SPK-CV-003"=FALSE, "SPK-CV-004"=FALSE, "SPK-CV-005"=FALSE, "SPK-CV-006"=FALSE, "SPK-CV-007"=FALSE, "SPK-CV-008"=FALSE, "SPW-CV-001"=FALSE, "SPW-CV-002"=FALSE, "SPW-CV-003"=FALSE, "SPW-CV-004"=FALSE, "SPW-CV-005"=FALSE, "SPW-CV-006"=FALSE, "SPW-CV-007"=FALSE, "SPW-CV-008"=FALSE, "SKM-CV-LAM"=FALSE, "SKM-CV-COR"=FALSE, "SKM-CV-JMP"=FALSE, "SKI-CV-AR"=FALSE, "SKI-CV-KF-ST"=FALSE, "SKI-CV-KF-BY1"=FALSE, "SKI-CV-WF-ST"=FALSE, "SKI-CV-WF-BY1"=FALSE, "SKI-CV-ST"=FALSE, "SKI-CV-BY2"=FALSE, "X31-27"=FALSE, "X31-28"=FALSE, "X31-29"=FALSE, "X31-30"=FALSE, "X31-31"=FALSE, "X31-32"=FALSE, "PID-PC-TQ-ON"=FALSE, "PID-FC-AR-ON"=FALSE, "PID-WF-ON"=FALSE, "PID-KF-ON"=FALSE, "PID-SA-WF-INV"=FALSE, "PID-SA-KF-INV"=FALSE, "PID-SA-AR-COR"=FALSE, "SPK-WR-ON"=FALSE, "SPW-WR-ON"=FALSE, "SPK-WR-OFF"=FALSE, "SPW-WR-OFF"=FALSE}, "ANALOGICO"={"SKM-PC-TQ"=0, "SKM-FC-AR"=0, "SKM-FC-WF"=0, "SKM-FC-KF"=0, "X33 5"=0, "X33 6"=0, "X33 7"=0, "X33 8"=0, "X33 9"=0, "X33 10"=0, "X33 11"=0, "X33 12"=0, "X33 13"=0, "X33 14"=0, "PID-PC-TQ-SP"=0, "PID-FC-AR-SP"=0, "PID-FC-WF-SP"=0, "PID-FC-KF-SP"=0, "PID-INC-WF-SP"=0, "PID-INC-KF-SP"=0, "SPK-WR-VEL"=0, "SPW-WR-VEL"=0, "SKM-FIC-COR-AR-MAX"=0.0, "SKM-FIC-COR-AR-MIN"=0.0, "SKM-FIC-COR-KF-MAX"=0.0, "SKM-FIC-COR-KF-MIN"=0.0, "PID-PC-TQ-GP"=0.0, "PID-PC-TQ-GI"=0.0, "PID-PC-TQ-GD"=0.0, "PID-FC-AR-GP"=0.0, "PID-FC-AR-GI"=0.0, "PID-FC-AR-GD"=0.0, "PID-FC-WF-GP"=0.0, "PID-FC-WF-GI"=0.0, "PID-FC-WF-GD"=0.0, "PID-FC-KF-GP"=0.0, "PID-FC-KF-GI"=0.0, "PID-FC-KF-GD"=0.0, "PID-INV-WF-GP"=0.0, "PID-INV-WF-GI"=0.0, "PID-INV-WF-GD"=0.0, "PID-INV-KF-GP"=0.0, "PID-INV-KF-GI"=0.0, "PID-INV-KF-GD"=0.0}}, "UCM.004.EEL.0200_SAIDA"={"DIGITAL"={"SKS-CV-001"=FALSE, "SKS-CV-002"=FALSE, "SKS-CV-003"=FALSE, "SKS-CV-004"=FALSE, "SKS-CV-005"=FALSE, "SKS-CV-006"=FALSE, "SHD-CV-001"=FALSE, "SHD-CV-002"=FALSE, "SHD-ON-OFF"=FALSE, "X31-10"=FALSE, "X31-11"=FALSE, "X31-12"=FALSE, "X31-13"=FALSE, "X31-14"=FALSE, "X31-15"=FALSE, "X31-16"=FALSE}, "ANALOGICO"={"GD-ST-ES"=0, "X33-2"=0}}, "INTERNO"={"DIGITAL"={"INTERNO-SI-SS-1"=FALSE, "INTERNO-SI-SS-2"=FALSE, "INTERNO-SI-SS-3"=FALSE, "INTERNO-SS-SW-1"=FALSE, "INTERNO-SS-SK-1"=FALSE, "INTERNO-SPW-SKM-1"=FALSE}, "ANALOGICO"={"INTERNO_RESERVA"=0.0}}}  # todos_os_dados_SAIDA
            # "Verifica se está no PC Server\nse estiver, roda pelo diretorio\nlocal"
            # "todos os dados iniciando como\ndefault, mas serão sobrescrito pelo server"
            # "Inicializacao das variaveis"
            n51 = local write "Status_Comunicação"("" ("Status")) -> ()
            n52 = local write "Erro"(errorcluster {"status"=FALSE, "code"=0, "source"=""} ("error constant")) -> ()
            n53 = local write "todos_os_dados_SAIDA"(w160) -> ()
            n54 = local write "todos_os_dados_ENTRADA"(w159) -> ()
            n55 = call "Meu_IP_Address.vi"() -> ("Meu IP"=w168:string)  [unwired: 4 in, 1 out]
            n56 = Equal?(x=w168, y="143.106.176.228") -> (x = y?=w166:bool)
            n57 = case shown="False" w166 {
              tunnel: ["143.106.170.228" ("Combo Box") "localhost" ("Combo Box")] -> w165
              frame False {
              }
              frame True {
              }
            }
            n58 = local write "Endereço IP do Server"(w165) -> ()
          }
        }
      }
      event "[ESC]": Value Change {
        w177 = T5 {"UCM.004.EEL.0300_ENTRADA"={"DIGITAL"={"X30 1"=FALSE, "X30 2"=FALSE, "X30 3"=FALSE, "X30 4"=FALSE, "X30 5"=FALSE, "X30 6"=FALSE, "X30 7"=FALSE, "X30 8"=FALSE, "X30 9"=FALSE, "X30 10"=FALSE, "X30 11"=FALSE, "X30 12"=FALSE, "X30 13"=FALSE, "X30 14"=FALSE, "X30 15"=FALSE, "X30 16"=FALSE, "SPK-RD-ALR"=FALSE, "SPK-RD-VVT"=FALSE, "SPK-RD-FLL"=FALSE, "SPW-RD-ALR"=FALSE, "SPW-RD-VVT"=FALSE, "SPW-RD-FLL"=FALSE}, "ANALOGICO"={"SKM-PA-BAR"=0, "SKM-PA-TQ"=0, "SKM-TI-TQ"=0, "SKM-PA-LAM"=0, "SKM-TI-LAM"=0, "SKM-PD-LAM"=0, "SKM-TI-WF"=0, "SKM-FIM-WF"=0, "SIT-PI-001"=0, "SKI-PD-ST"=0, "SIT-PI-MS1"=0, "SIT-PI-MS2"=0, "SKM-TI-KF"=0, "SPW-PD-P"=0, "SPK-PD-P"=0, "X32 16 "=0, "X32 17"=0, "X32 18"=0, "X32 19"=0, "X32 20"=0, "X32 21"=0, "X32 22"=0, "X32 23"=0, "X32 24"=0, "SPK-RD-ST"=0, "SPW-RD-ST"=0, "SPK-RD-VEL"=0, "SPW-RD-VEL"=0, "SPK-RD-IA"=0, "SPW-RD-IA"=0, "SPK-RD-TU"=0, "SPW-RD-TU"=0, "SKM-TI-COR-KF"=0.0, "SKM-DEN-COR-KF"=0.0, "SKM-FIC-COR-KF"=0.0, "SKM-TI-COR-AR"=0.0, "SKM-DEN-COR-AR"=0.0, "SPK-RD-CRT"=0.0, "SPW-RD-CRT"=0.0, "SKM-FIC-COR-AR"=0.0}}, "UCM.004.EEL.0200_ENTRADA"={"DIGITAL"={"SKS-LAH-S"=FALSE, "SKS-LAH-W"=FALSE, "SKS-LAH-K"=FALSE, "SKS-MIN-W"=FALSE, "SKS-MAX-W"=FALSE, "SKS-MIN-K"=FALSE, "SKS-MAX-K"=FALSE, "X30-8"=FALSE, "X30-9"=FALSE, "X30-10"=FALSE, "X30-11"=FALSE, "X30-12"=FALSE, "X30-13"=FALSE, "X30-14"=FALSE, "X30-15"=FALSE, "X30-16"=FALSE}, "ANALOGICO"={"SKS-LC-K"=0, "SKS-LC-W"=0, "SHD-TI-AMB"=0, "X32-4"=0, "SHD-PI-01"=0, "SHD-PI-02"=0, "SIT-PI-MS3"=0, "SIT-PI-03"=0}}, "INTERNO"={"DIGITAL"={"INTERNO-SI-SS-1"=FALSE, "INTERNO-SI-SS-2"=FALSE, "INTERNO-SI-SS-3"=FALSE, "INTERNO-SS-SW-1"=FALSE, "INTERNO-SS-SK-1"=FALSE, "INTERNO-SPW-SKM-1"=FALSE}, "ANALOGICO"={"INTERNO_RESERVA"=0.0}}}  # todos_os_dados_ENTRADA
        w178 = T1 {"UCM.004.EEL.0300_SAIDA"={"DIGITAL"={"SPK-CV-001"=FALSE, "SPK-CV-002"=FALSE, "SPK-CV-003"=FALSE, "SPK-CV-004"=FALSE, "SPK-CV-005"=FALSE, "SPK-CV-006"=FALSE, "SPK-CV-007"=FALSE, "SPK-CV-008"=FALSE, "SPW-CV-001"=FALSE, "SPW-CV-002"=FALSE, "SPW-CV-003"=FALSE, "SPW-CV-004"=FALSE, "SPW-CV-005"=FALSE, "SPW-CV-006"=FALSE, "SPW-CV-007"=FALSE, "SPW-CV-008"=FALSE, "SKM-CV-LAM"=FALSE, "SKM-CV-COR"=FALSE, "SKM-CV-JMP"=FALSE, "SKI-CV-AR"=FALSE, "SKI-CV-KF-ST"=FALSE, "SKI-CV-KF-BY1"=FALSE, "SKI-CV-WF-ST"=FALSE, "SKI-CV-WF-BY1"=FALSE, "SKI-CV-ST"=FALSE, "SKI-CV-BY2"=FALSE, "X31-27"=FALSE, "X31-28"=FALSE, "X31-29"=FALSE, "X31-30"=FALSE, "X31-31"=FALSE, "X31-32"=FALSE, "PID-PC-TQ-ON"=FALSE, "PID-FC-AR-ON"=FALSE, "PID-WF-ON"=FALSE, "PID-KF-ON"=FALSE, "PID-SA-WF-INV"=FALSE, "PID-SA-KF-INV"=FALSE, "PID-SA-AR-COR"=FALSE, "SPK-WR-ON"=FALSE, "SPW-WR-ON"=FALSE, "SPK-WR-OFF"=FALSE, "SPW-WR-OFF"=FALSE}, "ANALOGICO"={"SKM-PC-TQ"=0, "SKM-FC-AR"=0, "SKM-FC-WF"=0, "SKM-FC-KF"=0, "X33 5"=0, "X33 6"=0, "X33 7"=0, "X33 8"=0, "X33 9"=0, "X33 10"=0, "X33 11"=0, "X33 12"=0, "X33 13"=0, "X33 14"=0, "PID-PC-TQ-SP"=0, "PID-FC-AR-SP"=0, "PID-FC-WF-SP"=0, "PID-FC-KF-SP"=0, "PID-INC-WF-SP"=0, "PID-INC-KF-SP"=0, "SPK-WR-VEL"=0, "SPW-WR-VEL"=0, "SKM-FIC-COR-AR-MAX"=0.0, "SKM-FIC-COR-AR-MIN"=0.0, "SKM-FIC-COR-KF-MAX"=0.0, "SKM-FIC-COR-KF-MIN"=0.0, "PID-PC-TQ-GP"=0.0, "PID-PC-TQ-GI"=0.0, "PID-PC-TQ-GD"=0.0, "PID-FC-AR-GP"=0.0, "PID-FC-AR-GI"=0.0, "PID-FC-AR-GD"=0.0, "PID-FC-WF-GP"=0.0, "PID-FC-WF-GI"=0.0, "PID-FC-WF-GD"=0.0, "PID-FC-KF-GP"=0.0, "PID-FC-KF-GI"=0.0, "PID-FC-KF-GD"=0.0, "PID-INV-WF-GP"=0.0, "PID-INV-WF-GI"=0.0, "PID-INV-WF-GD"=0.0, "PID-INV-KF-GP"=0.0, "PID-INV-KF-GI"=0.0, "PID-INV-KF-GD"=0.0}}, "UCM.004.EEL.0200_SAIDA"={"DIGITAL"={"SKS-CV-001"=FALSE, "SKS-CV-002"=FALSE, "SKS-CV-003"=FALSE, "SKS-CV-004"=FALSE, "SKS-CV-005"=FALSE, "SKS-CV-006"=FALSE, "SHD-CV-001"=FALSE, "SHD-CV-002"=FALSE, "SHD-ON-OFF"=FALSE, "X31-10"=FALSE, "X31-11"=FALSE, "X31-12"=FALSE, "X31-13"=FALSE, "X31-14"=FALSE, "X31-15"=FALSE, "X31-16"=FALSE}, "ANALOGICO"={"GD-ST-ES"=0, "X33-2"=0}}, "INTERNO"={"DIGITAL"={"INTERNO-SI-SS-1"=FALSE, "INTERNO-SI-SS-2"=FALSE, "INTERNO-SI-SS-3"=FALSE, "INTERNO-SS-SW-1"=FALSE, "INTERNO-SS-SK-1"=FALSE, "INTERNO-SPW-SKM-1"=FALSE}, "ANALOGICO"={"INTERNO_RESERVA"=0.0}}}  # todos_os_dados_SAIDA
        # "Processo de parada, manda as variaveis para default e desliga, as variaveis vai para default apenas por uma questao de \"beleza\" quando o programa encerrar"
        n59 = event-data() -> ()  [unwired: 1 in, 1 out]
        n60 = local write "Erro"(errorcluster {"status"=FALSE, "code"=0, "source"=""} ("error constant")) -> ()
        n61 = local write "led_indica_comunicacao"(FALSE ("led_indica_comunicacao")) -> ()
        n62 = local write "Status_Comunicação"("VI Desligada:\n1) Antes de rodá-la, certifique-se que o Server esteja ligado\n2) Para executá-la aperte Ctrl+R" ("Status_Comunicação")) -> ()
        n63 = local write "todos_os_dados_ENTRADA"(w177) -> ()
        n64 = local write "todos_os_dados_SAIDA"(w178) -> ()
      }
    }
  }
  n65 = TCP Close Connection(connection ID=w10, error in (no error)=w9) -> (error out=w8:errorcluster)  [unwired: 1 in, 1 out]
  n66 = call <vilib>:"Clear Errors.vi"("error in (no error)"=w8) -> ()  [unwired: 5 in, 2 out]
  n67 = call <vilib>:"Close Config Data.vi"("error in (no error)"=w7, "refnum"=w6) -> ("error out"=w5:errorcluster)  [unwired: 8 in, 1 out]
  n68 = call <vilib>:"Clear Errors.vi"("error in (no error)"=w5) -> ()  [unwired: 5 in, 2 out]
